vi "Set Write Parameters.vi"(0 "Transaction":T2=enum."RFFE-Ext Write", 5 "Wait Ticks":u32, 7 "Bytes to Write":u8, 9 "Socket Mask [U32]":u32 format="%06x", 11 "error in (no error)":errorcluster, 14 "FPGA":T1) -> (15 "error out":errorcluster)   [LabVIEW 2017, in "Host SRL.lvlib"]
uses:
  Host SRL.lvlib
  Type Defs/WSVCAP SHL Transaction Enum.ctl
  Type Defs/WSVCAP SHL FPGA Enum.ctl
  Type Defs/WSVCAP SHL Top Level Control Operation Enum.ctl
  Type Defs/WSVCAP SHL State.ctl
  Type Defs/WSVCAP SHL Top Level Control Enum.ctl
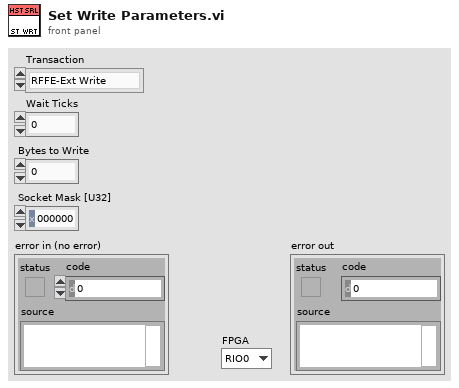
[diagram p1: front panel]
types:
  T1 = typedef "WSVCAP SHL FPGA Enum.ctl" = enum16{"RIO0", "RIO1"}
  T2 = typedef "WSVCAP SHL Transaction Enum.ctl" = enum16{"I2C-Read Data", "I2C-Write Data", "RFFE-Ext Write", "RFFE-Ext Read", "SRL-Write Data"}
  T3 = typedef "WSVCAP SHL Top Level Control Operation Enum.ctl" = enum16{"Initialize", "Set Control", "Read Control", "Close"}
  T4 = typedef "WSVCAP SHL State.ctl" = enum8{"Idle", "Transfer Data"}
  T5 = typedef "WSVCAP SHL Top Level Control Enum.ctl" = enum16{"Start", "Cmd", "Transaction", "Wait Ticks", "Socket Mask", "UUT Set", "Slave Address", "Sub Address", "Bytes to Write", "Bytes to Read", "Write Data", "Write Flag", "Read Data", "Read Flag", "Ack Read", "Read Status Flag", "Ack Read Status", "Status", "Cycle Count", "Stop Cycle", "Exit"}
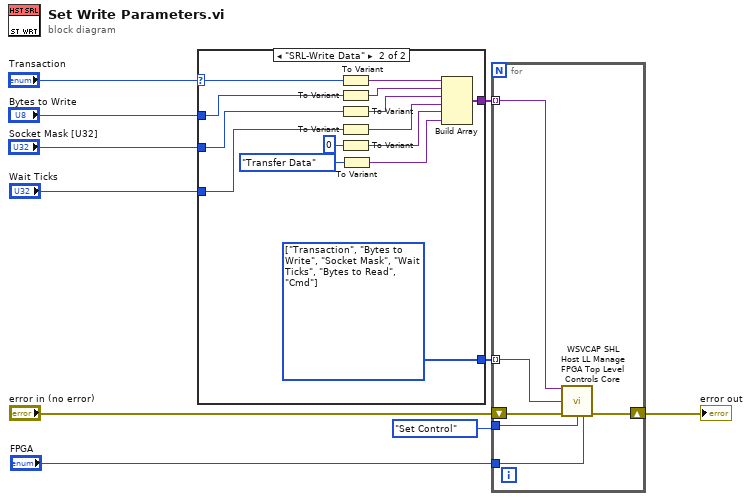
[diagram p0: block diagram]
diagram:
  n1 = case shown="\"SRL-Write Data\"" "Transaction" {
    selector: "Transaction" -> [_ w13]
    tunnel: [_ w21] -> w9
    tunnel: [_ w19] -> w6
    tunnel: "Socket Mask [U32]" -> [_ w18]
    tunnel: "Bytes to Write" -> [_ w16]
    tunnel: "Wait Ticks" -> [_ w15]
    frame Default {
    }
    frame "SRL-Write Data" {
      w19 = T5[] [enum."Transaction", enum."Bytes to Write", enum."Socket Mask", enum."Wait Ticks", enum."Bytes to Read", enum."Cmd"] items=["Start", "Cmd", "Transaction", "Wait Ticks", "Socket Mask", "UUT Set", "Slave Address", "Sub Address", "Bytes to Write", "Bytes to Read", "Write Data", "Write Flag", "Read Data", "Read Flag", "Ack Read", "Read Status Flag", "Ack Read Status", "Status", "Cycle Count", "Stop Cycle", "Exit"]
      n2 = To Variant(anything=w13) -> (Variant=w23:variant)
      n3 = To Variant(anything=w16) -> (Variant=w22:variant)
      n4 = To Variant(anything=w18) -> (Variant=w17:variant)
      n5 = To Variant(anything=w15) -> (Variant=w14:variant)
      n6 = To Variant(anything=u8 0 ("Bytes to Read (Ext-Read Only)")) -> (Variant=w12:variant)
      n7 = To Variant(anything=WSVCAP_SHL_State."Transfer Data" ("SPI_Cmd")) -> (Variant=w20:variant)
      n8 = Build Array(w23, w22, w17, w14, w12, w20) -> (w21:variant[])
    }
  }
  n9 = for {
    tunnel: WSVCAP_SHL_Top_Level_Control_Operation_Enum."Set Control" ("Operation") -> [w30]
    tunnel: w9 -> [w29] mode=indexing
    tunnel: w6 -> [w28] mode=indexing
    shift-right: [w26] -> w7
    shift-left: "error in (no error)" -> [w27]
    tunnel: "FPGA" -> [w25]
    n10 = call "WSVCAP SHL Host LL Manage FPGA Top Level Controls Core.vi"("Value In"=w29, "FPGA Top Level Control"=w28, "error in (no error)"=w27, "Operation"=w30, "FPGA"=w25) -> ("error out"=w26:errorcluster)  [unwired: 9 in, 1 out]
  }
  "error out" <- w7
